vi "setAaf.vi"(0 "connection ID":refnum<k5>, 1 "enable":bool=TRUE, 2 "attenuation":i32, 3 "window":i32, 5 "error":errorcluster) -> (14 "connection ID out":refnum<k5>, 19 "error out":errorcluster)   [LabVIEW 2016, in "sen_api.lvlib"]
doc: "Sets the anti-aliasing filter with assigned filter window."
uses:
  sen_api.lvlib
panel:
  out "jsonRespIn":string
  out "JSON-response":string="{\"jsonrpc\":\"2.0\",\"method\":\"\",\"params\":[5,1.245,true,\"name\"],\"id\":\"1\"}"
  out "JSON request":string
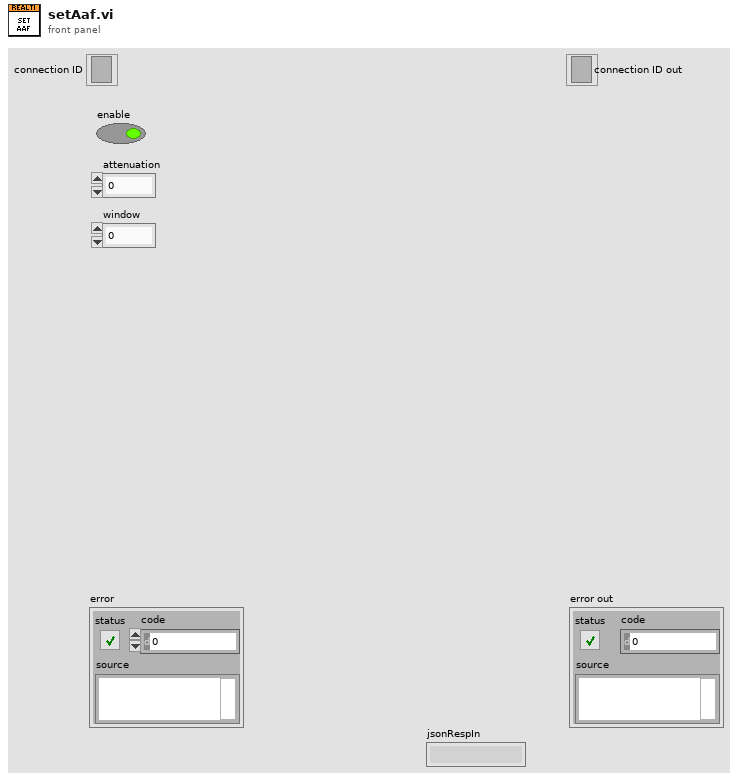
[diagram p1: front panel]
types:
  T1 = cluster{"jsonrpc":string, "method":string, "params":string[], "id":string, "api":i32, "pid":string}
  T2 = enum16{"Standard", "Buffered", "CRLF", "Immediate"}
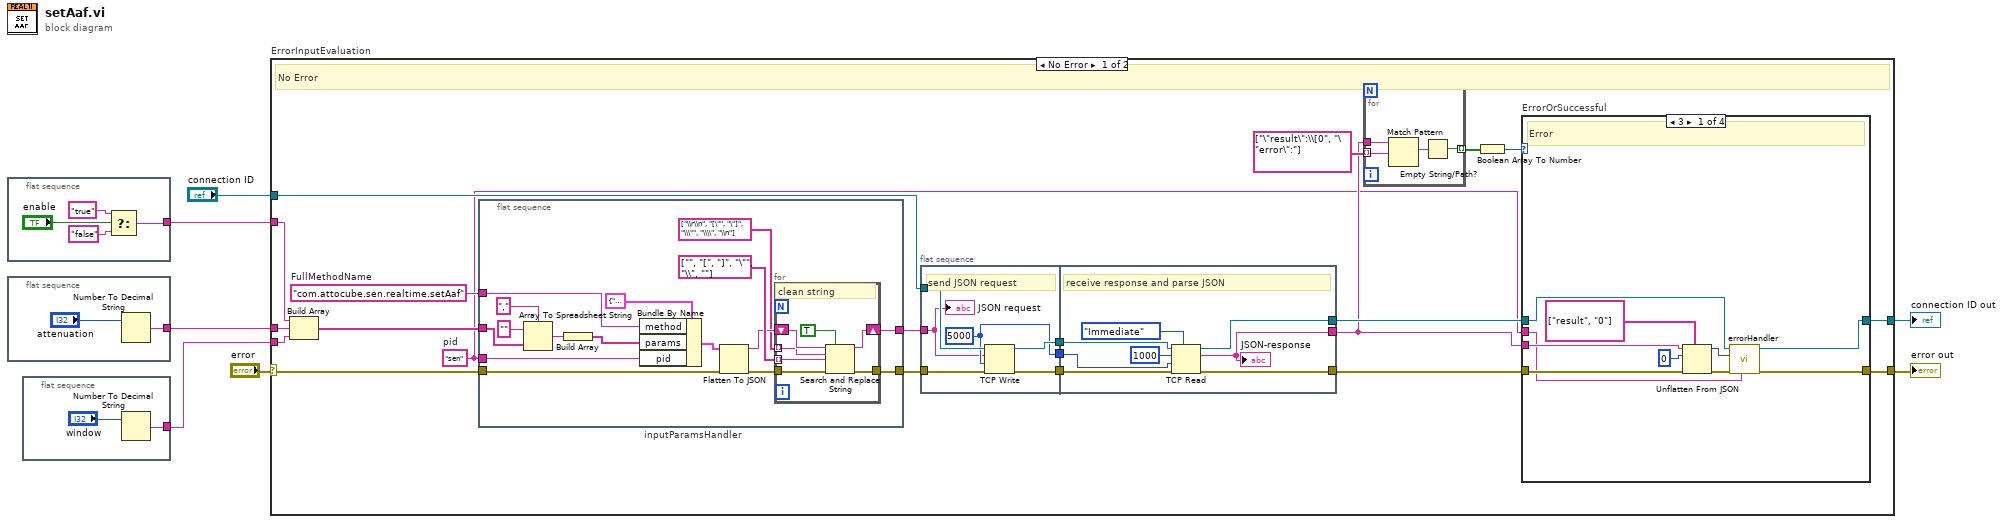
[diagram p0: block diagram]
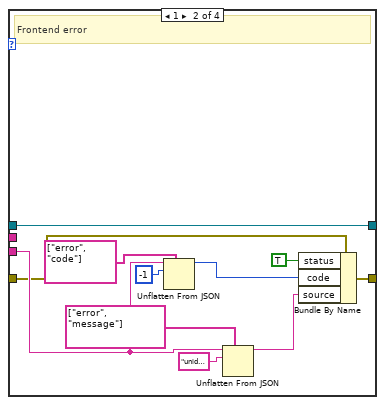
[diagram p2: hidden frame]
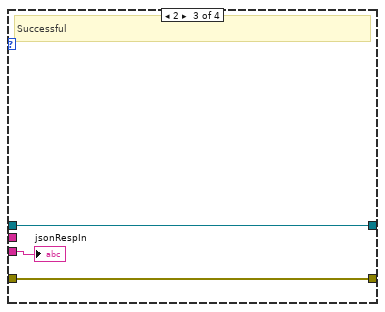
[diagram p3: hidden frame]
diagram:
  n1 = flat-sequence "in_bool" {
    tunnel: [w8] -> w3
    frame #0 {
      n2 = Select(t="true" ("Base"), s="enable", f="false" ("Base")) -> (s? t:f=w8:string)
    }
  }
  n3 = flat-sequence "in_integer" {
    tunnel: [w12] -> w2
    frame #0 {
      n4 = Number To Decimal String(number="attenuation") -> (decimal integer string=w12:string)  [unwired: 1 in]
    }
  }
  n5 = flat-sequence "in_integer" {
    tunnel: [w14] -> w1
    frame #0 {
      n6 = Number To Decimal String(number="window") -> (decimal integer string=w14:string)  [unwired: 1 in]
    }
  }
  n7 = case "ErrorInputEvaluation" shown="No Error" "error" {
    selector: "error" -> [w29 w104]
    tunnel: "connection ID" -> [w33 w105]
    tunnel: [w20 w104] -> w6
    tunnel: [w21 w105] -> w5
    tunnel: w3 -> [w18 _]
    tunnel: w2 -> [w17 _]
    tunnel: w1 -> [w16 _]
    frame No Error {
      w19 = "sen"  # pid
      w30 = "com.attocube.sen.realtime.setAaf"  # FullMethodName
      # "No Error"
      n8 = Build Array ("ParametersArrayString")(w18, w17, w16) -> (w28:string[])
      n9 = flat-sequence "inputParamsHandler" {
        tunnel: [w66] -> w27
        tunnel: w28 -> [w73]
        tunnel: w29 -> [w71]
        tunnel: [w68] -> w26
        tunnel: w30 -> [w74]
        tunnel: w19 -> [w63]
        frame #0 {
          n10 = Array To Spreadsheet String(delimiter (Tab)=",", array=w73, 3:"" ("format string")) -> (spreadsheet string=w76:string)
          n11 = Build Array "Build Array"(w76) -> (w72:string[])
          n12 = Bundle By Name(cluster=T1 {"jsonrpc"="2.0", "method"="com.attocube.amc.res.setRESReadOutFreq", "params"=[], "id"="1", "api"=2, "pid"=""} ("Cluster"), "method"=w74, "params"=w72, "pid"=w63) -> (w75:T1)
          n13 = Flatten To JSON(anything=w75, error in (no error)=w71) -> (JSON string=w67:string, 11:w69:errorcluster)  [unwired: 1 in]
          n14 = for {
            tunnel: string[] ["\\r\\n", "[\"", "\"]", "\\\"", "\\\\", "\\n"] ("search string") -> [w82] mode=indexing
            tunnel: string[] ["", "[", "]", "\"", "\\", ""] ("replace string (\"\")") -> [w81] mode=indexing
            shift-right: [w84] -> w66
            shift-left: w67 -> [w83]
            tunnel: w69 -> [w80]
            tunnel: [w79] -> w68
            # "clean string"
            n15 = Search and Replace String(replace all?=TRUE ("replace all? (F)"), input string=w83, search string=w82, replace string=w81, error in=w80) -> (result string=w84:string, error out=w79:errorcluster)  [unwired: 3 in, 2 out]
          }
        }
      }
      n16 = flat-sequence {
        tunnel: w33 -> [w95]
        tunnel: [w93] -> w36
        tunnel: [w94] -> w35
        tunnel: w26 -> [w90]
        tunnel: [w92] -> w34
        tunnel: w27 -> [w91]
        tunnel: [w99] -> w25
        tunnel: w36 -> [w101]
        tunnel: w35 -> [w100]
        tunnel: [w97] -> w24
        tunnel: w34 -> [w98]
        tunnel: [w96] -> w23
        frame #0 {
          w92 = 5000 ("timeout ms (25000)")
          # "send JSON request"
          n17 = TCP Write(connection ID=w95, data in=w91, error in (no error)=w90, 9:w92) -> (connection ID out=w93:refnum<k5>, error out=w94:errorcluster)  [unwired: 1 out]
          "JSON request" <- w91
        }
        frame #1 {
          # "receive response and parse JSON"
          n18 = TCP Read(connection ID=w101, bytes to read=1000, error in (no error)=w100, 7:T2."Immediate" ("mode (standard)"), 9:w98) -> (connection ID out=w99:refnum<k5>, data out=w96:string, error out=w97:errorcluster)
          "JSON-response" <- w96
        }
      }
      n19 = for {
        tunnel: string[] ["\"result\":\\[0", "\"error\":"] ("path") -> [w88] mode=indexing
        tunnel: [w86] -> w31 mode=indexing
        tunnel: w23 -> [w89]
        n20 = Match Pattern(string=w89, regular expression=w88) -> (match substring=w87:string)  [unwired: 1 in, 3 out]
        n21 = Empty String/Path?(string/path=w87) -> (empty?=w86:bool)
      }
      n22 = Boolean Array To Number(Boolean array=w31) -> (number=w22:u32)
      n23 = case "ErrorOrSuccessful" shown="3" w22 {
        tunnel: w23 -> [w40 w49 w58 _]
        tunnel: w25 -> [w44 w47 w60 w62]
        tunnel: [w42 w47 w60 w62] -> w21
        tunnel: [w43 w50 w59 w61] -> w20
        tunnel: w24 -> [w46 w48 w59 w61]
        tunnel: w19 -> [w37 _ _ _]
        frame 3 {
          # "Error"
          n24 = Unflatten From JSON(path=string[] ["result", "0"], JSON string=w40, type and defaults=0, error in (no error)=w46) -> (value=w38:i32, error out=w45:errorcluster)  [unwired: 3 in]
          n25 = call "errorHandler.vi"("pid"=w37, "error in"=w45, "errNbr"=w38, "connection ID"=w44) -> ("error out 2"=w43:errorcluster, "connection ID out"=w42:refnum<k5>)  [unwired: 6 in]
        }
        frame 1 {
          # "Frontend error"
          n26 = Unflatten From JSON(path=string[] ["error", "code"], JSON string=w49, type and defaults=-1) -> (value=w56:i32)  [unwired: 4 in, 1 out]
          n27 = Unflatten From JSON(path=string[] ["error", "message"], JSON string=w49, type and defaults="unidentified error") -> (value=w57:string)  [unwired: 4 in, 1 out]
          n28 = Bundle By Name(cluster=w48, "status"=TRUE, "code"=w56, "source"=w57) -> (w50:errorcluster)
        }
        frame 2 {
          # "Successful"
          "jsonRespIn" <- w58
        }
        frame Default {
          # "NoResponse"
        }
      }
    }
    frame Error {
      # "Error"
    }
  }
  "error out" <- w6
  "connection ID out" <- w5
